vi "DC Bus Test_TS_BB_v3.vi"(8 "error in (no error)":errorcluster, 11 "Control Board VISA":refnum<visa-resource-name>) -> (0 "error out":errorcluster, 3 "Inv_DC":dbl[](array[numeric]))   [LabVIEW 2022 SP3]
uses:
  Serial Board Com/ADCSelector BB.ctl
panel:
  out "INV B (0V)":dbl
  out "INV A (0V)":dbl
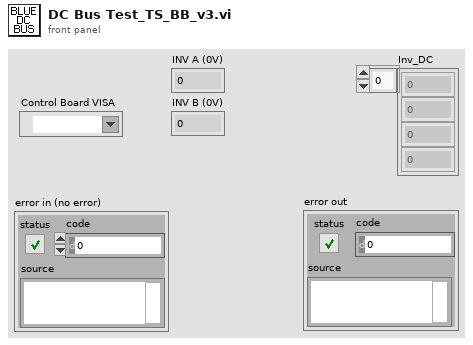
[diagram p1: front panel]
types:
  T1 = typedef "ADCSelector BB.ctl" = enum16{"INVA_ISENSE_U", "INVA_ISENSE_V", "INVA_ISENSE_W", "INVA_UDC", "INVA_TEMP", "HB_TEMP", "AUXB_TEMP", "VLINE_AB", "VLINE_BC", "VLINE_CA", "VSENSE_POS_24V", "VSENSE_POS_5V", "VSENSE_NEG_15V", "INVB_ISENSE_U", "INV_B_ISENSEV", "INVB_ISENSE_W", "INVB_UDC", "INVB_TEMP", "AUXA_TEMP", "AUXC_TEMP", "VOUT_AB", "VOUT_BC", "VOUT_CA", "VSENSE_POS_15V", "VSENSE_POS_3P3V", "TEST_POINT"}
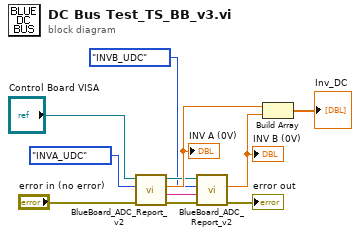
[diagram p0: block diagram]
diagram:
  n1 = call "BlueBoard_ADC_Report_v2.vi"("error in (no error)"="error in (no error)", "Blue Board Enum"=ADCSelector_BB."INVA_UDC", "ControlBoard VISA"="Control Board VISA") -> ("error out"=w11:errorcluster, "Message OUT"=w10:string, "Result"=w7:dbl, "VISA Refnum out"=w3:refnum<visa-resource-name>)  [unwired: 5 in]
  "INV A (0V)" <- w7
  n2 = call "BlueBoard_ADC_Report_v2.vi"("error in (no error)"=w11, "Message IN"=w10, "Blue Board Enum"=ADCSelector_BB."INVB_UDC", "ControlBoard VISA"=w3) -> ("error out"=→"error out":errorcluster, "Result"=w6:dbl)  [unwired: 4 in, 2 out]
  "INV B (0V)" <- w6
  n3 = Build Array(w7, w6) -> (→"Inv_DC":dbl[])
